vi "写入量程参数.vi"(8 "error in (no error)":errorcluster, 10 "自动测试量程配置":T2={"水样测试量程模式"=enum."H", "标样核查量程模式"=enum."H", "零点核查量程模式"=enum."H", "跨度核查量程模式"=enum."H", "空白测试量程模式"=enum."H", "平行样测试量程模式"=enum."H", "加标回收量程模式"=enum."H"}, 11 "MB session in":refnum<class "MB_Master.lvclass">) -> (0 "error out":errorcluster, 3 "MB session out":refnum<class "MB_Master.lvclass">)   [LabVIEW 2016, in "斯坦道CODMn新电路板.lvlib"]
uses:
  <vilib>/Plasmionique/MB Master/MB_Master/MB_Master.lvclass
  <vilib>/Plasmionique/MB Master/MB_Master_Serial/MB_Master_Serial.lvclass
  D:/Program Files (x86)/National Instruments/LabVIEW 2016/vi.lib/Plasmionique/MB Master/MB_Master/MB_Master.lvclass
  <vilib>/Plasmionique/MB Master/MB Master.lvlib
panel:
  in  "VISA Resource":refnum<visa-resource-name>
  in  "引用选择":enum16{"MB引用", "自建引用"}(ring)
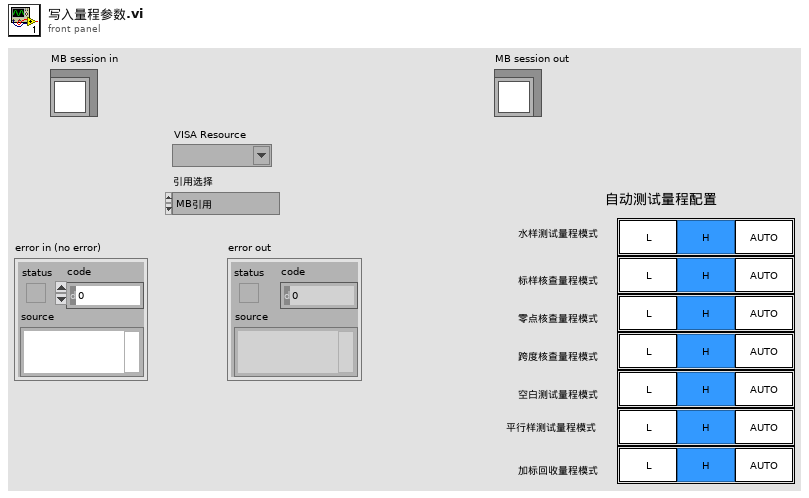
[diagram p1: front panel]
types:
  T1 = typedef "量程选择控件.ctl" = enum32{"L", "H", "AUTO"}
  T2 = cluster{"水样测试量程模式":T1, "标样核查量程模式":T1, "零点核查量程模式":T1, "跨度核查量程模式":T1, "空白测试量程模式":T1, "平行样测试量程模式":T1, "加标回收量程模式":T1}
  T3 = cluster{"baud rate (bps)":u32, "stop bits":u16, "parity":u16, "flow control":u16, "timeout":u32, "retries":i32}
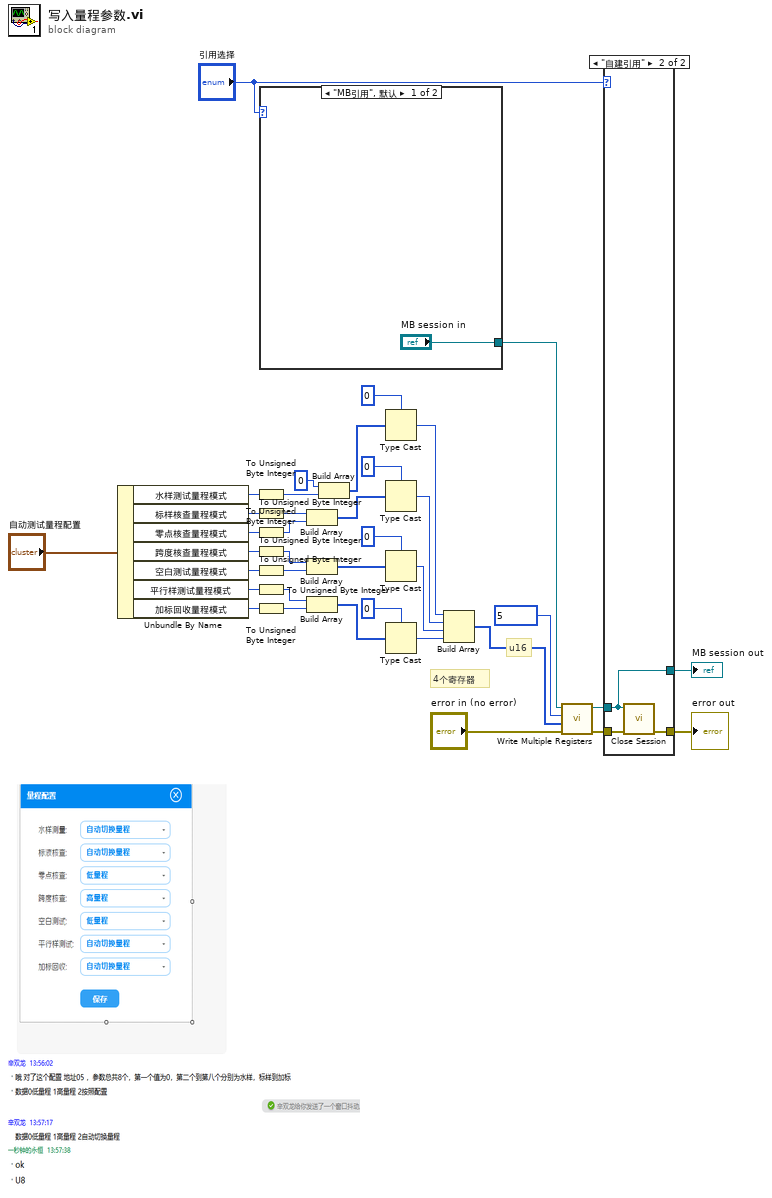
[diagram p0: block diagram]
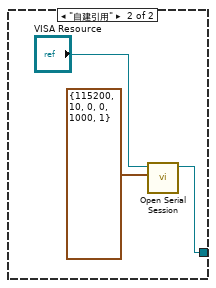
[diagram p3: hidden frame]
diagram:
  # "4个寄存器"
  # "u16"
  n1 = Unbundle By Name("自动测试量程配置") -> ("水样测试量程模式"=w14:T1, "标样核查量程模式"=w12:T1, "零点核查量程模式"=w10:T1, "跨度核查量程模式"=w8:T1, "空白测试量程模式"=w7:T1, "平行样测试量程模式"=w5:T1, "加标回收量程模式"=w4:T1)
  n2 = To Unsigned Byte Integer(number=w14) -> (unsigned 8bit integer=w13:u8)
  n3 = To Unsigned Byte Integer(number=w12) -> (unsigned 8bit integer=w11:u8)
  n4 = To Unsigned Byte Integer(number=w10) -> (unsigned 8bit integer=w9:u8)
  n5 = To Unsigned Byte Integer(number=w8) -> (unsigned 8bit integer=w2:u8)
  n6 = To Unsigned Byte Integer(number=w7) -> (unsigned 8bit integer=w1:u8)
  n7 = To Unsigned Byte Integer(number=w5) -> (unsigned 8bit integer=w6:u8)
  n8 = To Unsigned Byte Integer(number=w4) -> (unsigned 8bit integer=w3:u8)
  n9 = case shown="\"MB引用\", 默认" "引用选择" {
    tunnel: ["MB session in" w41] -> w35
    frame "MB引用", Default {
    }
    frame "自建引用" {
      n10 = call <vilib>:"Open Serial Session.vi"("Serial Config"=T3 {"baud rate (bps)"=115200, "stop bits"=10, "parity"=0, "flow control"=0, "timeout"=1000, "retries"=1}, "VISA Resource"="VISA Resource") -> ("MB_Serial session"=w41:refnum<class "MB_Master_Serial.lvclass">)  [unwired: 8 in, 1 out]
    }
  }
  n11 = Build Array(w11, w9) -> (w27:u8[])
  n12 = Build Array(w2, w1) -> (w17:u8[])
  n13 = Build Array(w6, w3) -> (w22:u8[])
  n14 = Build Array(u8 0, w13) -> (w28:u8[])
  n15 = Type Cast(type=u16 0, x=w28) -> (*(type *) &x=w24:u16)
  n16 = Type Cast(type=u16 0, x=w27) -> (*(type *) &x=w23:u16)
  n17 = Type Cast(type=u16 0, x=w17) -> (*(type *) &x=w16:u16)
  n18 = Type Cast(type=u16 0, x=w22) -> (*(type *) &x=w15:u16)
  n19 = Build Array(w24, w23, w16, w15) -> (w25:u16[])
  n20 = call <vilib>:"Write Multiple Registers.vi"("error in (no error)"="error in (no error)", "values"=w25, "starting address"=u16 5, "MB session in"=w35) -> ("error out"=w32:errorcluster, "MB session out"=w34:refnum<class "MB_Master.lvclass">)  [unwired: 6 in]
  n21 = case shown="\"自建引用\"" "引用选择" {
    tunnel: w34 -> [w42 w44]
    tunnel: w32 -> [w43 w46]
    tunnel: [w43 w45] -> w31
    tunnel: [w42 w44] -> w30
    frame "MB引用", Default {
    }
    frame "自建引用" {
      n22 = call-dynamic "Close Session.vi"("error in (no error)"=w46, "MB session in"=w44) -> ("error out"=w45:errorcluster)  [unwired: 9 in]
    }
  }
  "MB session out" <- w30
  "error out" <- w31
